vi "Read Identifier.vi"(8 "error in":errorcluster, 11 "Ballard ARINC-429 Execution Unit in":refnum<class "Ballard ARINC-429 Execution Unit.lvclass">) -> (0 "error out":errorcluster, 2 "identifier":string, 3 "Ballard ARINC-429 Execution Unit out":refnum<class "Ballard ARINC-429 Execution Unit.lvclass">)   [LabVIEW 2020, in "Ballard ARINC 429 Engine.lvlib" / "Implementation.lvlib" / "Ballard ARINC-429 Execution Unit.lvclass"]
uses:
  Ballard ARINC-429 Execution Unit.lvclass
  Ballard ARINC-429 Execution Unit.lvclass/Ballard ARINC-429 Execution Unit.ctl
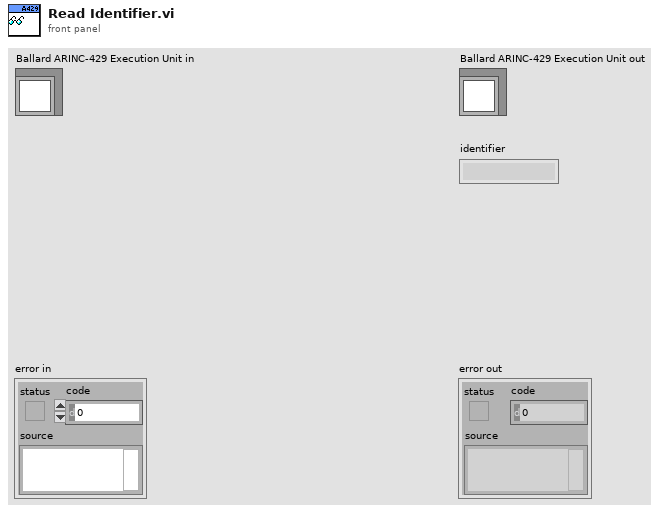
[diagram p1: front panel]
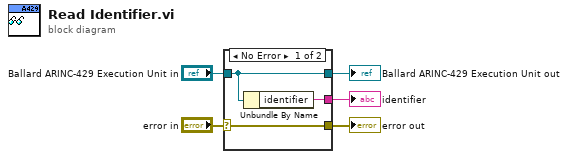
[diagram p0: block diagram]
diagram:
  n1 = case shown="No Error" "error in" {
    selector: "error in" -> [w8 w9]
    tunnel: [w8 w9] -> w4
    tunnel: [w7 w10] -> w2
    tunnel: "Ballard ARINC-429 Execution Unit in" -> [w7 w10]
    tunnel: [w6 _] -> w1
    frame No Error {
      n2 = Unbundle By Name(w7) -> ("identifier"=w6:string)
    }
    frame Error {
    }
  }
  "error out" <- w4
  "Ballard ARINC-429 Execution Unit out" <- w2
  "identifier" <- w1
